vi "Create.vi"(8 "error in (no error)":errorcluster, 10 "PWM module":T1=enum."PWM1", 11 "connection ID":i32=-1) -> (0 "error out":errorcluster, 3 "MicroDAQ.lvlib:PWM.lvclass":refnum<class "PWM.lvclass">)   [LabVIEW 2009, in "MicroDAQ.lvlib" / "PWM.lvclass"]
uses:
  <instrlib>/MicroDAQ/Channel/PWM/PWM.lvclass
  <instrlib>/MicroDAQ/Tools/PWM channel.ctl
  <instrlib>/MicroDAQ/Channel/PWM/PWM.lvclass/PWM.ctl
  <instrlib>/MicroDAQ/Mlink library wraper/mlink.lvlib
  <instrlib>/MicroDAQ/Channel/Channel.lvclass
  <instrlib>/MicroDAQ/MicroDAQ.lvlib
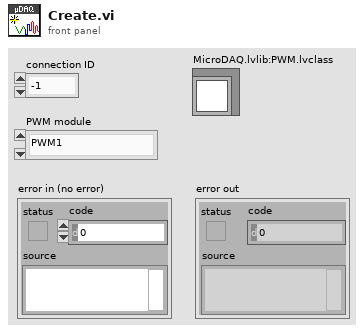
[diagram p1: front panel]
types:
  T1 = typedef "MicroDAQ.lvlib/PWM channel.ctl" = enum8{"None", "PWM1", "PWM2", "PWM3"}
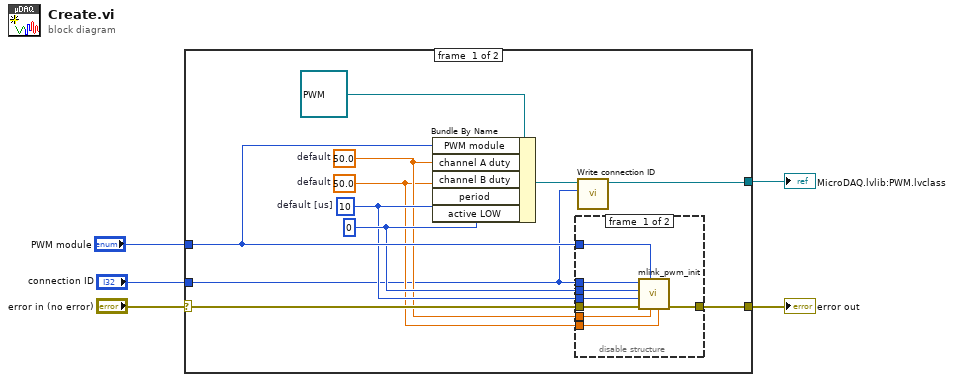
[diagram p0: block diagram]
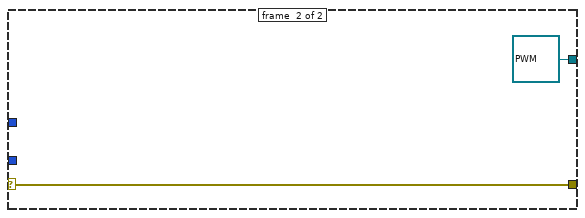
[diagram p3: hidden frame]
diagram:
  n1 = case shown="No Error" "error in (no error)" {
    selector: "error in (no error)" -> [w14 w27]
    tunnel: [w16 w27] -> w4
    tunnel: "connection ID" -> [w6 _]
    tunnel: "PWM module" -> [w13 _]
    tunnel: [w7 refnum<class "PWM.lvclass"> refnum ("MicroDAQ.lvlib:PWM.lvclass")] -> w1
    frame #0 {
      w12 = u8 0 ("active LOW")
      w11 = u32 10  # default [us]
      w9 = sgl 50.0  # default
      w10 = sgl 50.0  # default
      n2 = Bundle By Name(cluster=refnum<class "PWM.lvclass"> refnum ("MicroDAQ.lvlib:PWM.lvclass"), "PWM module"=w13, "channel A duty"=w10, "channel B duty"=w9, "period"=w11, "active LOW"=w12) -> (w8:refnum<class "PWM.lvclass">)
      n3 = disable-structure shown="Enabled" {
        disable-tunnel: [w24 w25] -> w16
        disable-tunnel: w14 -> [w23 w25]
        disable-tunnel: w6 -> [w22 _]
        disable-tunnel: w13 -> [w21 _]
        disable-tunnel: w12 -> [w20 _]
        disable-tunnel: w11 -> [w19 _]
        disable-tunnel: w10 -> [w18 _]
        disable-tunnel: w9 -> [w17 _]
        frame #0 {
          n4 = call <instrlib>:"mlink_pwm_init.vi"("channel B duty"=w17, "channel A duty"=w18, "PWM module"=w21, "error in (no error)"=w23, "period"=w19, "active LOW"=w20, "connection ID"=w22) -> ("error out"=w24:errorcluster)  [unwired: 3 in, 1 out]
        }
        frame #1 {
          # "test"
        }
      }
      n5 = call <instrlib>:"Write connection ID.vi"("connection ID"=w6, "Task in"=w8) -> ("Task out"=w7:refnum<class "PWM.lvclass">)  [unwired: 9 in]
    }
    frame #1 {
    }
  }
  "error out" <- w4
  "MicroDAQ.lvlib:PWM.lvclass" <- w1
